vi "Convert to POV Direction.vi"(11 "POVs in":i16[](array[numeric])) -> (3 "POV Direction":T1)   [LabVIEW 2023, in "GameController_SEN.lvlib"]
uses:
  GameController_SEN.lvlib
  Type Defs/ENUM_POV_Direction.ctl
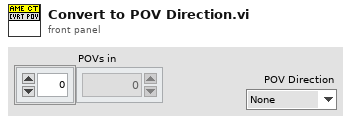
[diagram p1: front panel]
types:
  T1 = typedef "ENUM_POV_Direction.ctl" = enum16{"None", "Up", "UpRight", "Right", "DownRight", "Down", "DownLeft", "Left", "UpLeft"}
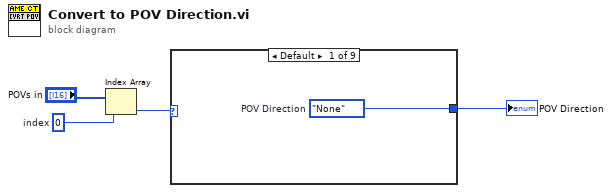
[diagram p0: block diagram]
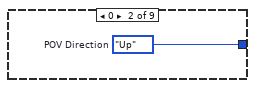
[diagram p2: hidden frame]
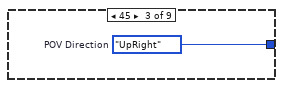
[diagram p3: hidden frame]
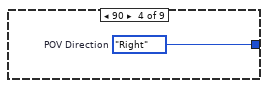
[diagram p4: hidden frame]
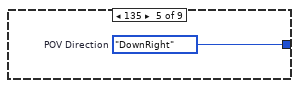
[diagram p5: hidden frame]
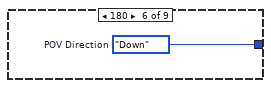
[diagram p6: hidden frame]
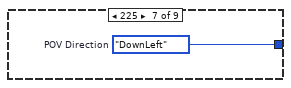
[diagram p7: hidden frame]
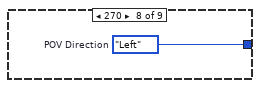
[diagram p8: hidden frame]
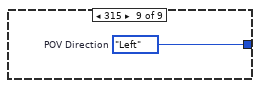
[diagram p9: hidden frame]
diagram:
  w3 = 0  # index
  n1 = Index Array(array="POVs in", index=w3) -> (element=w2:i16)
  n2 = case shown="Default" w2 {
    tunnel: [w5 w6 w7 w8 w9 w10 w11 w12 w13] -> w1
    frame Default {
      w5 = ENUM_POV_Direction."None"  # POV Direction
    }
    frame 0 {
      w6 = ENUM_POV_Direction."Up"  # POV Direction
    }
    frame 45 {
      w7 = ENUM_POV_Direction."UpRight"  # POV Direction
    }
    frame 90 {
      w8 = ENUM_POV_Direction."Right"  # POV Direction
    }
    frame 135 {
      w9 = ENUM_POV_Direction."DownRight"  # POV Direction
    }
    frame 180 {
      w10 = ENUM_POV_Direction."Down"  # POV Direction
    }
    frame 225 {
      w11 = ENUM_POV_Direction."DownLeft"  # POV Direction
    }
    frame 270 {
      w12 = ENUM_POV_Direction."Left"  # POV Direction
    }
    frame 315 {
      w13 = ENUM_POV_Direction."Left"  # POV Direction
    }
  }
  "POV Direction" <- w1
